vi "Stations.Overview.vi"() -> ()   [LabVIEW 2015, in "Stations.Overview.lvlib"]
uses:
  Stations.Overview.lvlib
  Types/Overview.StateVariables.ctl
  Types/Overview.Channels.ctl
  <vilib>/NI Veristand/Execution/Workspace/SystemStateEventRef.ctl
  <vilib>/NI Veristand/Execution/Workspace/Target State Info.ctl
  <vilib>/NI Veristand/Execution/Workspace/Target State.ctl
  <vilib>/NI Veristand/Execution/Workspace/WorkspaceAPI.ctl
  Execution GUI/Types/Execute.UserEventRefs.ctl
  <vilib>/NI Veristand/Execution/Workspace/SystemStateRegEventRef.ctl
  <vilib>/NI Veristand/Execution/WaveformStreaming/Waveform Data Watcher Event Data (DBL).ctl
  <vilib>/NI Veristand/Execution/WaveformStreaming/WaveformStreamSpecification.ctl
  <vilib>/NI/AMC/Read Termination Message.vi
  <vilib>/NI/AMC/Update Message Routing Info.vi
  <vilib>/NI/AMC/Create Multiple Messages.vi
  <vilib>/NI/AMC/Create Single Message.vi
  <vilib>/NI/AMC/Globals.vi
  <vilib>/NI/AMC/Send Message.vi
  <vilib>/NI/AMC/AMC.lvlib
  <vilib>/NI Veristand/Execution/Workspace/NI_VS Workspace ExecutionAPI.lvlib
  Execution GUI/Station.Execution.lvlib
  NationalInstruments.VeriStand.ClientAPI
  <vilib>/NI Veristand/Execution/WaveformStreaming/NI_VS Waveform Streaming Interface.lvlib
panel:
  in  "Station.IDs":string[](array[string])=["DUT1"]
  in  "NIVS.Gateway IP Address":string="localhost"
  in  "NIVS.Workspace Event":refnum<event-registration>
  out "Station ID":string
  out "Multicolumn Listbox":i32(listbox)
  in  "Station.ID":string="All"
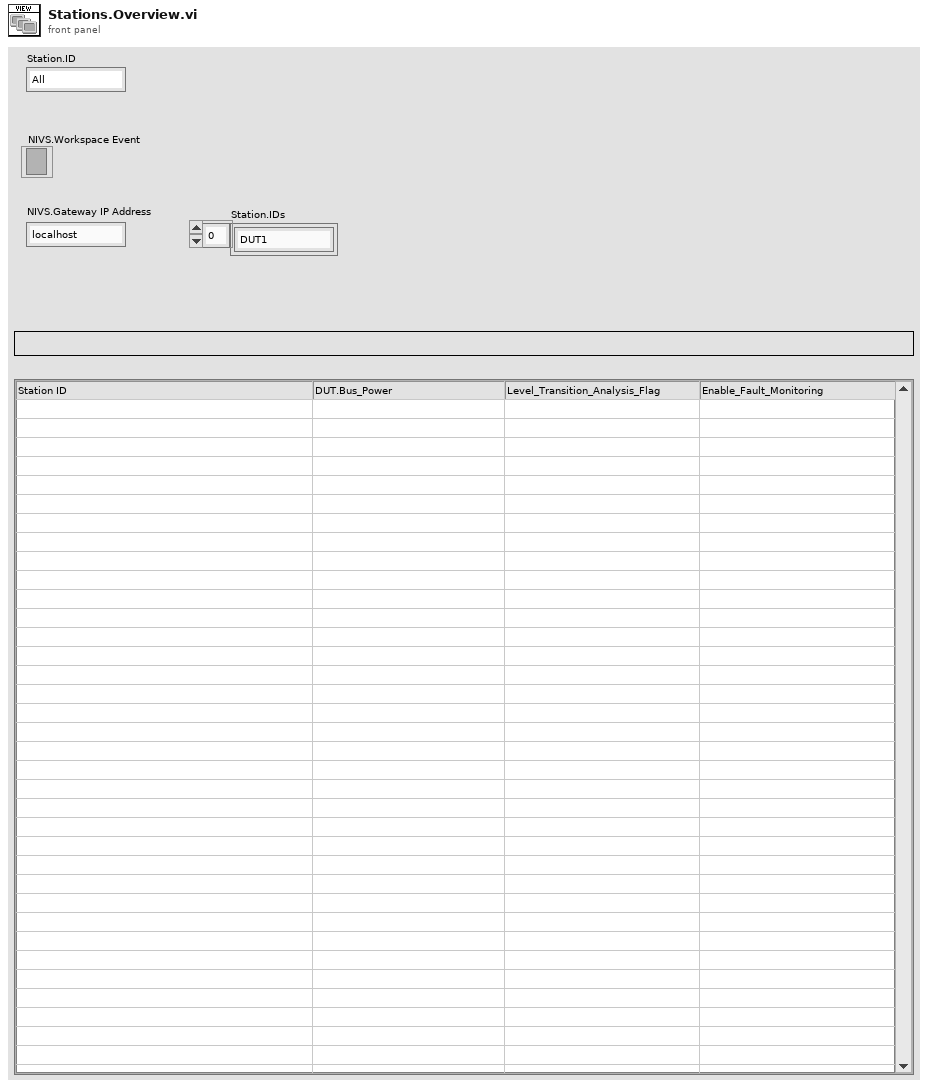
[diagram p1: front panel]
types:
  T1 = typedef "Stations.Overview.lvlib/Overview.StateVariables.ctl" = cluster{"UI.Table":refnum<vi>, "Channel.List":T2[], "Station.IDs":string[], "NIVS.SystemStateRefs":T3, "NIVS.WorkspaceManager":T4, "NIVS.Deployed":bool, "NIVS.GatewayIPAddress":string, "NIVS.Events":T5, "NIVS.SystemDefinitionFile":path, "NIVS.Open":bool}
  T2 = typedef "Stations.Overview.lvlib/Overview.Channels.ctl" = cluster{"Channel.List":string[]}
  T3 = typedef "NI_VS Workspace ExecutionAPI.lvlib/SystemStateEventRef.ctl" = cluster{"CustDatRef":refnum<user-event>, "EvtRef":refnum<k27>, "Target State User Event":refnum<user-event>}
  T4 = typedef "NI_VS Workspace ExecutionAPI.lvlib/WorkspaceAPI.ctl" = refnum<k24>
  T5 = typedef "Station.Execution.lvlib/Execute.UserEventRefs.ctl" = cluster{"SystemChangeEvent":T6, "WorkspaceEvent":refnum<event-registration>, "WaveformEvent":refnum<event-registration>}
  T6 = typedef "NI_VS Workspace ExecutionAPI.lvlib/SystemStateRegEventRef.ctl" = refnum<event-registration>
  T7 = typedef "AMC.lvlib/Message Queue.ctl" = refnum<queue>
  T8 = typedef "NI_VS Workspace ExecutionAPI.lvlib/SystemState.ctl" = u8
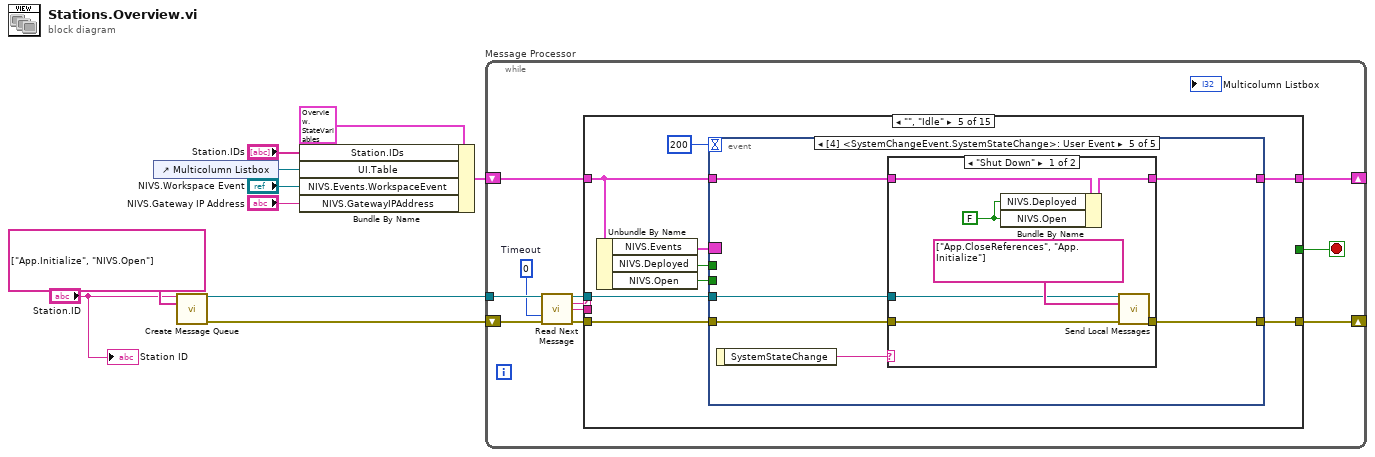
[diagram p0: block diagram]
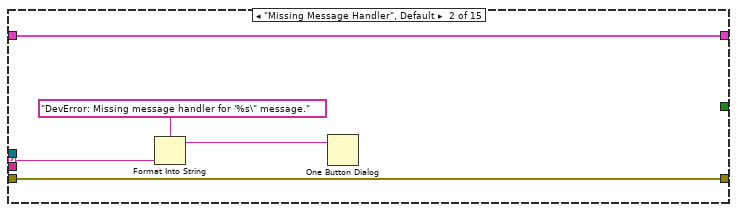
[diagram p3: hidden frame]
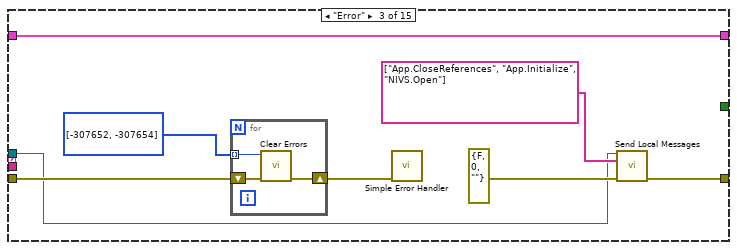
[diagram p4: hidden frame]
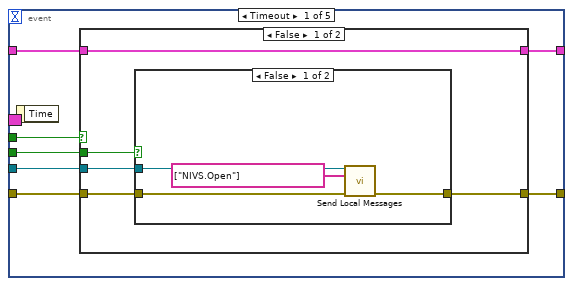
[diagram p6: hidden frame]
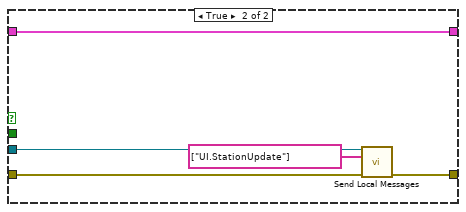
[diagram p8: hidden frame]
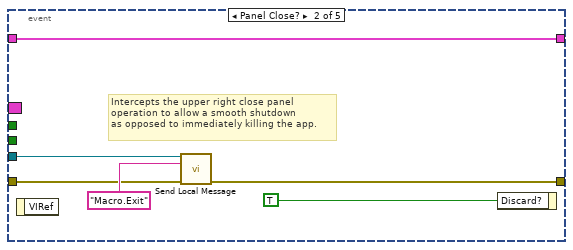
[diagram p9: hidden frame]
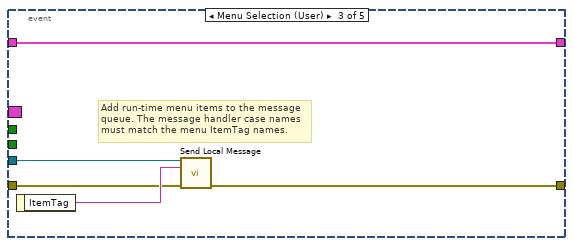
[diagram p10: hidden frame]
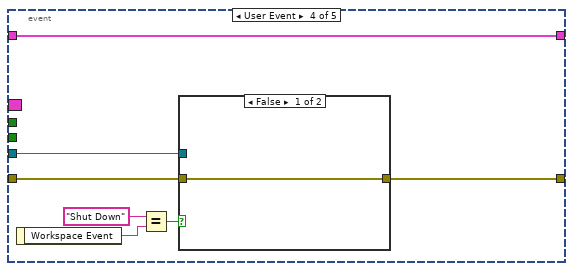
[diagram p11: hidden frame]
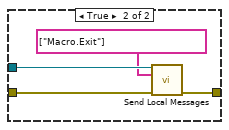
[diagram p12: hidden frame]
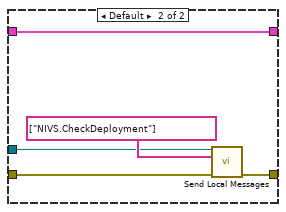
[diagram p13: hidden frame]
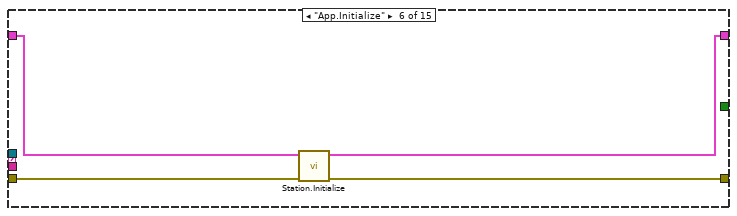
[diagram p14: hidden frame]
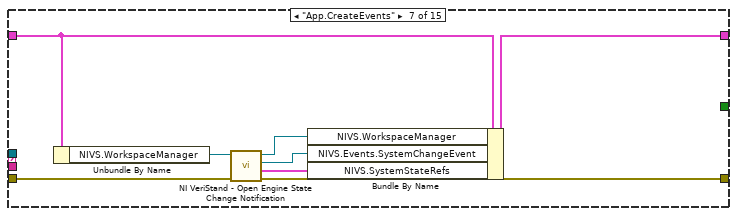
[diagram p15: hidden frame]
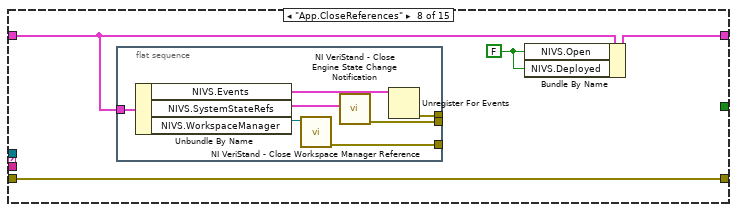
[diagram p16: hidden frame]
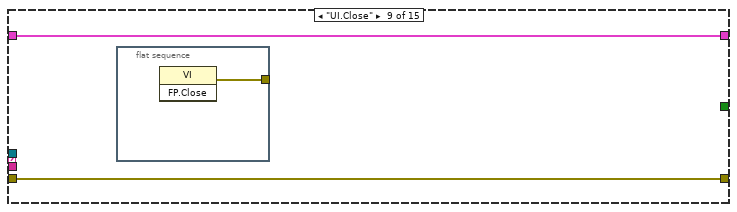
[diagram p17: hidden frame]
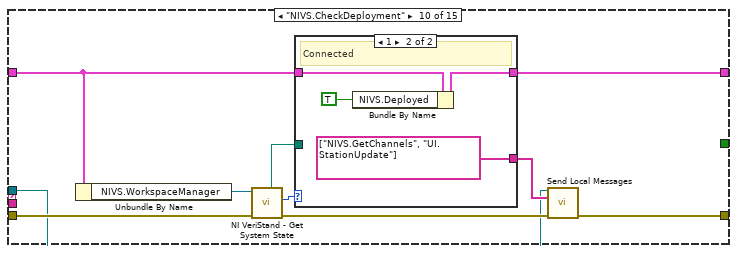
[diagram p18: hidden frame]
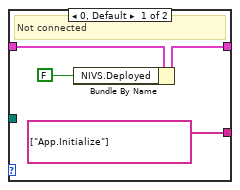
[diagram p19: hidden frame]
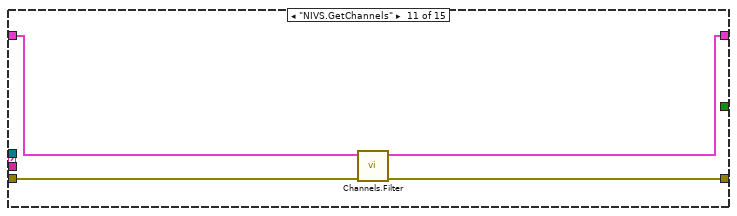
[diagram p20: hidden frame]
diagram:
  n1 = control-ref of="Multicolumn Listbox"() -> (w6:refnum<vi>)
  n2 = call <vilib>:"Create Message Queue.vi"("message queue name"="Station.ID", "initial message names"=string[] ["App.Initialize", "NIVS.Open"]) -> ("message queue out"=w9:T7, "error out"=w1:errorcluster)  [unwired: 12 in]
  n3 = Bundle By Name(cluster=T1 {"UI.Table"=refnum, "Channel.List"=[], "Station.IDs"=[], "NIVS.SystemStateRefs"={"CustDatRef"=refnum, "EvtRef"=refnum, "Target State User Event"=refnum}, "NIVS.WorkspaceManager"=refnum, "NIVS.Deployed"=FALSE, "NIVS.GatewayIPAddress"="", "NIVS.Events"={"SystemChangeEvent"=refnum, "WorkspaceEvent"=refnum, "WaveformEvent"=refnum}, "NIVS.SystemDefinitionFile"=path "", "NIVS.Open"=FALSE} ("state variables"), "Station.IDs"="Station.IDs", "UI.Table"=w6, "NIVS.Events.WorkspaceEvent"="NIVS.Workspace Event", "NIVS.GatewayIPAddress"="NIVS.Gateway IP Address") -> (w7:T1)
  n4 = while "Message Processor" {
    shift-left: w1 -> [w16]
    shift-right: [w19] -> _
    tunnel: w9 -> [w17]
    shift-left: w7 -> [w21]
    shift-right: [w20] -> _
    stop <- w11 stop-if-true
    w12 = 0  # Timeout
    n5 = call <vilib>:"Read Next Message.vi"("message queue in"=w17, "timeout (1 ms)"=w12, "error in"=w16) -> ("message queue out"=w18:T7, "message name"=w14:string, "message value"=w13:string, "error out"=w15:errorcluster)  [unwired: 5 in, 4 out]
    n6 = case shown="\"\", \"Idle\"" w14 {
      selector: w14 -> [_ w26 _ _ _ _ _ _ _ _ _ _ _ _ _]
      tunnel: [w23 w28 w36 w41 w43 w116 w121 w127 w137 w141 w158 w167 w182 w189 w194] -> w20
      tunnel: w21 -> [w23 w28 w36 w41 w44 w117 w120 w128 w137 w142 w159 w165 w182 w189 w194]
      tunnel: w18 -> [_ _ w29 _ w50 _ _ _ _ w143 _ w163 _ w185 w192]
      tunnel: w15 -> [w22 w27 w34 w40 w49 w115 w125 w129 w138 w144 w161 w166 w184 w187 w193]
      tunnel: [w22 w27 w30 w40 w48 w114 w124 w129 w138 w140 w160 w162 w183 w186 w191] -> w19
      tunnel: w13 -> [_ _ _ _ _ _ _ _ _ _ _ _ _ _ _]
      tunnel: [_ _ _ _ _ _ _ _ _ _ _ _ _ _ TRUE] -> w11
      frame "---------- Framework Operations ----------" {
      }
      frame "Missing Message Handler", Default {
        n7 = Format Into String(format string="DevError: Missing message handler for '%s\" message." ("message"), w26) -> (resulting string=w24:string)  [unwired: 2 in, 1 out]
        n8 = One Button Dialog(message=w24) -> ()  [unwired: 2 out]
      }
      frame "Error" {
        n9 = for {
          shift-right: [w38] -> w35
          shift-left: w34 -> [w39]
          tunnel: i32[] [-307652, -307654] -> [w37] mode=indexing
          n10 = call <vilib>:"Clear Errors.vi"("error in (no error)"=w39, "specific error code to clear (0: all)"=w37) -> ("error out"=w38:errorcluster)  [unwired: 4 in, 1 out]
        }
        n11 = call <vilib>:"Simple Error Handler.vi"("error in (no error)"=w35) -> ()  [unwired: 1 in, 8 out]
        n12 = call <vilib>:"Send Local Messages.vi"("message queue in"=w29, "message names"=string[] ["App.CloseReferences", "App.Initialize", "NIVS.Open"], "error in"=errorcluster {"status"=FALSE, "code"=0, "source"=""} ("error out")) -> ("error out"=w30:errorcluster)  [unwired: 10 in, 2 out]
      }
      frame "---------- Application Operations ----------" {
      }
      frame "", "Idle" {
        n13 = Unbundle By Name(w44) -> ("NIVS.Events"=w47:T5, "NIVS.Deployed"=w45:bool, "NIVS.Open"=w42:bool)
        n14 = event shown="[4] <SystemChangeEvent.SystemStateChange>: User Event" {
          selector: w47 -> [_ _ _ _ _]
          dyn-events: _ -> [_ _ _ _ _]
          timeout: 200 -> [_ _ _ _ _]
          tunnel: w50 -> [w57 w76 w82 w87 w99]
          tunnel: w49 -> [w56 w75 w81 w88 w100]
          tunnel: [w55 w74 w80 w86 w96] -> w48
          tunnel: w45 -> [w54 _ _ _ _]
          tunnel: w44 -> [w53 w73 w79 w85 w98]
          tunnel: [w52 w73 w79 w85 w97] -> w43
          tunnel: w42 -> [w51 _ _ _ _]
          event Timeout {
            n15 = event-data() -> ()  [unwired: 2 out]
            n16 = case shown="False" w54 {
              tunnel: w57 -> [w58 w72]
              tunnel: w56 -> [w60 w71]
              tunnel: [w59 w70] -> w55
              tunnel: w53 -> [w62 w68]
              tunnel: [w62 w68] -> w52
              tunnel: w51 -> [w61 _]
              frame False {
                n17 = case shown="False" w61 {
                  tunnel: w60 -> [w65 w67]
                  tunnel: [w64 w67] -> w59
                  tunnel: w58 -> [w63 _]
                  frame False {
                    n18 = call <vilib>:"Send Local Messages.vi"("message queue in"=w63, "message names"=string[] ["NIVS.Open"], "error in"=w65) -> ("error out"=w64:errorcluster)  [unwired: 10 in, 2 out]
                  }
                  frame True {
                  }
                }
              }
              frame True {
                n19 = call <vilib>:"Send Local Messages.vi"("message queue in"=w72, "message names"=string[] ["UI.StationUpdate"], "error in"=w71) -> ("error out"=w70:errorcluster)  [unwired: 10 in, 2 out]
              }
            }
          }
          event Panel Close? {
            # "Intercepts the upper right close panel\noperation to allow a smooth shutdown\nas opposed to immediately killing the app."
            n20 = event-data() -> ()  [unwired: 2 out]
            n21 = call <vilib>:"Send Local Message.vi"("message queue in"=w76, "message name"="Macro.Exit", "error in"=w75) -> ("error out"=w74:errorcluster)  [unwired: 10 in, 2 out]
            n22 = event-data("Discard?"=TRUE) -> ()  [unwired: 1 in, 1 out]
          }
          event Menu Selection (User) {
            # "Add run-time menu items to the message\nqueue. The message handler case names must match the menu ItemTag names."
            n23 = event-data() -> ("ItemTag"=w83:string)  [unwired: 1 out]
            n24 = call <vilib>:"Send Local Message.vi"("message queue in"=w82, "message name"=w83, "error in"=w81) -> ("error out"=w80:errorcluster)  [unwired: 10 in, 2 out]
          }
          event User Event {
            n25 = event-data() -> ("Workspace Event"=w84:string)  [unwired: 1 out]
            n26 = Equal?(x="Shut Down" ("y"), y=w84) -> (x = y?=w89:bool)
            n27 = case shown="False" w89 {
              tunnel: w88 -> [w91 w95]
              tunnel: [w91 w94] -> w86
              tunnel: w87 -> [_ w93]
              frame False {
              }
              frame True {
                n28 = call <vilib>:"Send Local Messages.vi"("message queue in"=w93, "message names"=string[] ["Macro.Exit"], "error in"=w95) -> ("error out"=w94:errorcluster)  [unwired: 10 in, 2 out]
              }
            }
          }
          event User Event {
            n29 = event-data() -> ("SystemStateChange"=w101:string)  [unwired: 1 out]
            n30 = case shown="\"Shut Down\"" w101 {
              tunnel: w100 -> [w107 w112]
              tunnel: w99 -> [w106 w111]
              tunnel: [w105 w110] -> w96
              tunnel: w98 -> [w104 w109]
              tunnel: [w103 w109] -> w97
              frame "Shut Down" {
                w102 = FALSE ("NIVS.Open")
                n31 = Bundle By Name(cluster=w104, "NIVS.Deployed"=w102, "NIVS.Open"=w102) -> (w103:T1)
                n32 = call <vilib>:"Send Local Messages.vi"("message queue in"=w106, "message names"=string[] ["App.CloseReferences", "App.Initialize"], "error in"=w107) -> ("error out"=w105:errorcluster)  [unwired: 10 in, 2 out]
              }
              frame Default {
                n33 = call <vilib>:"Send Local Messages.vi"("message queue in"=w111, "message names"=string[] ["NIVS.CheckDeployment"], "error in"=w112) -> ("error out"=w110:errorcluster)  [unwired: 10 in, 2 out]
              }
            }
          }
        }
      }
      frame "App.Initialize" {
        n34 = call "Station.Initialize.vi"("error in (no error)"=w115, "state variables in"=w117) -> ("error out"=w114:errorcluster, "state variables out"=w116:T1)  [unwired: 8 in]
      }
      frame "App.CreateEvents" {
        n35 = Unbundle By Name(w120) -> ("NIVS.WorkspaceManager"=w119:T4)
        n36 = call <vilib>:"NI VeriStand - Open Engine State Change Notification.vi"("error in (no error)"=w125, "WorkspaceManager in"=w119) -> ("error out"=w124:errorcluster, "SystemStateRefs"=w123:T3, "SystemChangeEventRef"=w122:T6, "WorkspaceManager out"=w118:T4)  [unwired: 6 in]
        n37 = Bundle By Name(cluster=w120, "NIVS.WorkspaceManager"=w118, "NIVS.Events.SystemChangeEvent"=w122, "NIVS.SystemStateRefs"=w123) -> (w121:T1)
      }
      frame "App.CloseReferences" {
        w126 = FALSE ("NIVS.Open")
        n38 = flat-sequence {
          tunnel: [w133] -> _
          tunnel: [w132] -> _
          tunnel: [w131] -> _
          tunnel: w128 -> [w130]
          frame #0 {
            n39 = Unbundle By Name(w130) -> ("NIVS.Events"=w136:T5, "NIVS.SystemStateRefs"=w135:T3, "NIVS.WorkspaceManager"=w134:T4)
            n40 = call <vilib>:"NI VeriStand - Close Workspace Manager Reference.vi"("WorkspaceManager"=w134) -> ("error out"=w131:errorcluster)  [unwired: 10 in]
            n41 = call <vilib>:"NI VeriStand - Close Engine State Change Notification.vi"("SystemStateRefs"=w135) -> ("error out"=w132:errorcluster)  [unwired: 10 in]
            n42 = Unregister For Events(event registration refnum=w136) -> (error out=w133:errorcluster)  [unwired: 1 in]
          }
        }
        n43 = Bundle By Name(cluster=w128, "NIVS.Open"=w126, "NIVS.Deployed"=w126) -> (w127:T1)
      }
      frame "UI.Close" {
        n44 = flat-sequence {
          tunnel: [w139] -> _
          frame #0 {
            n45 = invoke class="VI" method="FP.Close"() -> (error out=w139:errorcluster)  [unwired: 3 in, 2 out]
          }
        }
      }
      frame "NIVS.CheckDeployment" {
        n46 = Unbundle By Name(w142) -> ("NIVS.WorkspaceManager"=w146:T4)
        n47 = call <vilib>:"NI VeriStand - Get System State.vi"("error in (no error)"=w144, "WorkspaceManager in"=w146) -> ("error out"=w148:errorcluster, "System State"=w145:T8, "System Definition File"=w147:path)  [unwired: 5 in, 2 out]
        n48 = case shown="1" w145 {
          tunnel: w142 -> [w153 w157]
          tunnel: [w152 w155] -> w141
          tunnel: w147 -> [_ _]
          tunnel: [string[] ["App.Initialize"] string[] ["NIVS.GetChannels", "UI.StationUpdate"]] -> w149
          frame 0, Default {
            # "Not connected"
            n49 = Bundle By Name(cluster=w153, "NIVS.Deployed"=FALSE ("Connected")) -> (w152:T1)
          }
          frame 1 {
            # "Connected"
            n50 = Bundle By Name(cluster=w157, "NIVS.Deployed"=TRUE ("Connected")) -> (w155:T1)
          }
        }
        n51 = call <vilib>:"Send Local Messages.vi"("message queue in"=w143, "message names"=w149, "error in"=w148) -> ("error out"=w140:errorcluster)  [unwired: 10 in, 2 out]
      }
      frame "NIVS.GetChannels" {
        n52 = call "Channels.Filter.vi"("error in (no error)"=w161, "state variables in"=w159) -> ("error out"=w160:errorcluster, "state variables out"=w158:T1)  [unwired: 8 in]
      }
      frame "NIVS.Open" {
        n53 = Unbundle By Name(w165) -> ("NIVS.GatewayIPAddress"=w164:string)
        n54 = call <vilib>:"NI VeriStand - Open Workspace Manager Reference.vi"("Gateway IP Address (\"\": localhost)"=w164) -> ("error out"=w168:errorcluster, "WorkspaceManager"=w169:T4)  [unwired: 9 in]
        n55 = case shown="No Error" w168 {
          tunnel: w165 -> [w177 w180]
          tunnel: w169 -> [w176 _]
          tunnel: [w174 w179] -> w167
          tunnel: w166 -> [w173 w181]
          tunnel: [w172 w181] -> w162
          tunnel: w163 -> [w171 _]
          frame No Error {
            n56 = Bundle By Name(cluster=w177, "NIVS.Open"=TRUE, "NIVS.WorkspaceManager"=w176) -> (w174:T1)
            n57 = call <vilib>:"Send Local Messages.vi"("message queue in"=w171, "message names"=string[] ["App.CreateEvents", "NIVS.CheckDeployment"], "error in"=w173) -> ("error out"=w172:errorcluster)  [unwired: 10 in, 2 out]
          }
          frame Error {
            n58 = Bundle By Name(cluster=w180, "NIVS.Open"=FALSE) -> (w179:T1)
          }
        }
      }
      frame "UI.StationUpdate" {
        n59 = call "UI.StationUpdate.vi"("error in (no error)"=w184, "state variables"=w182) -> ("error out"=w183:errorcluster)  [unwired: 9 in]
      }
      frame "Macro.Exit" {
        n60 = call <vilib>:"Send Local Messages.vi"("message queue in"=w185, "message names"=string[] ["App.CloseReferences", "UI.Close", "App.Exit"], "error in"=w187) -> ("error out"=w186:errorcluster)  [unwired: 10 in, 2 out]
      }
      frame "App.Exit" {
        n61 = call <vilib>:"Destroy Message Queue.vi"("message queue in"=w192, "error in"=w193) -> ("error out"=w191:errorcluster)  [unwired: 11 in, 2 out]
      }
    }
  }
  "Station ID" <- "Station.ID"
